vi "Progress.vi"(9 "iteration":i32, 10 "Message":string, 11 "Stop":bool) -> (3 "stop":bool)   [LabVIEW 2018]
doc: "Use this template to create a dialog box. This template polls the state of the buttons on the front panel and does not use events. Use the Dialog Using Events template (not available in the Base package) to create a dialog box with event handling."
panel:
  out "String 2":string
  out "Slide":u8(slide) scale=0.0..100.0
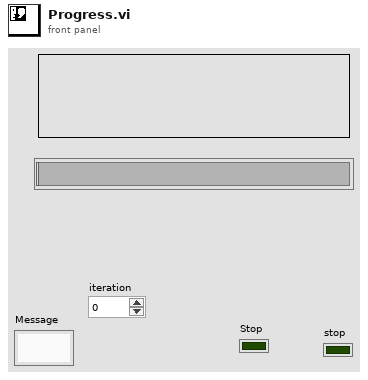
[diagram p1: front panel]
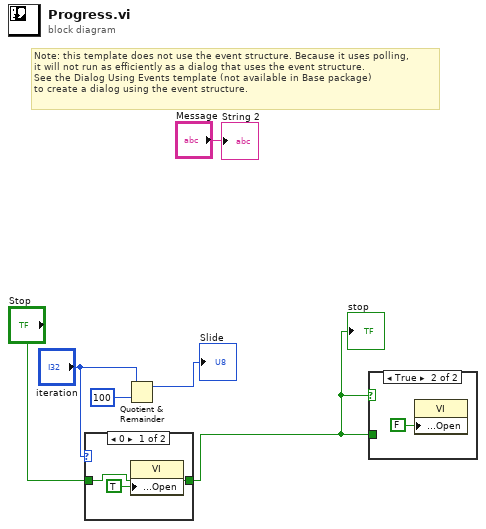
[diagram p0: block diagram]
diagram:
  # "Note: this template does not use the event structure. Because it uses polling, \nit will not run as efficiently as a dialog that uses the event structure.\nSee the Dialog Using Events template (not available in Base package) \nto create a dialog using the event structure."
  n1 = case shown="0" "iteration" {
    tunnel: "Stop" -> [w7 w9]
    tunnel: [w7 w9] -> w1
    frame 0 {
      n2 = property class="VI"("Front Panel.Open"=TRUE ("Front Panel Window:Open")) -> ()  [unwired: 2 in, 2 out]
    }
    frame 1, Default {
    }
  }
  "stop" <- w1
  n3 = Quotient & Remainder(x="iteration", y=100) -> (x-y*floor(x/y)=→"Slide":i32)  [unwired: 1 out]
  n4 = case shown="True" w1 {
    tunnel: w1 -> [_ _]
    frame False {
    }
    frame True {
      n5 = property class="VI"("Front Panel.Open"=FALSE ("Front Panel Window:Open")) -> ()  [unwired: 2 in, 2 out]
    }
  }
  "String 2" <- "Message"
